vi "TCP Server Templates - VI Tree.vi"   [LabVIEW 2020, in "JKI TCP Server.lvclass"]
uses:
  JKI TCP Server.lvclass
panel:
  # "OpenGOOP Templates VI Tree\nSee Diagram"
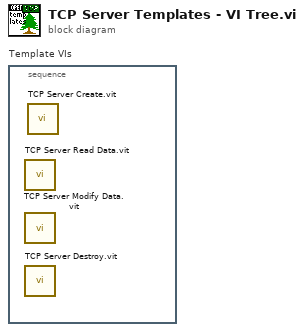
[diagram p0: block diagram]
diagram:
  n1 = stacked-sequence "Template VIs" {
    frame #0 {
      n2 = call "TCP Server Read Data.vit"() -> ()  [unwired: 10 in, 2 out]
      n3 = call "TCP Server Modify Data.vit"() -> ()  [unwired: 10 in, 2 out]
      n4 = call "TCP Server Destroy.vit"() -> ()  [unwired: 11 in, 1 out]
      n5 = call "TCP Server Create.vit"() -> ()  [unwired: 10 in, 2 out]
    }
  }
